vi "CI-recieveStatus.vi"(8 "error in (no error)":errorcluster, 10 "status":T1, 11 "common-interface in":refnum<class "VG-VNA_GUI.lvclass">) -> (0 "error out":errorcluster, 3 "common-interface out":refnum<class "VG-VNA_GUI.lvclass">)   [LabVIEW 2020, in "VG-VNA_GUI.lvlib" / "VG-VNA_GUI.lvclass"]
uses:
  VG-VNA_GUI.lvclass
  common/interface/CI-common_interface/CI-status_clust.ctl
  common/interface/CI-common_interface/CI-module_enum.ctl
  common/interface/CI-common_interface/CI-common_interface.lvclass
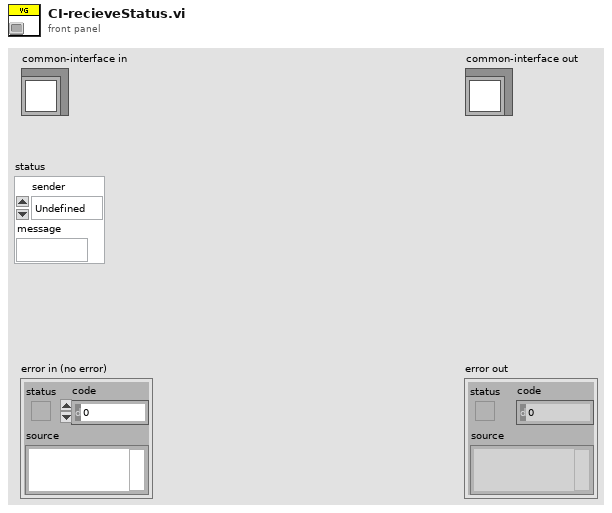
[diagram p1: front panel]
types:
  T1 = typedef "CI-common_interface.lvlib/CI-common_interface.lvclass/CI-status_clust.ctl" = cluster{"sender":T2, "message":string}
  T2 = typedef "CI-common_interface.lvlib/CI-common_interface.lvclass/CI-module_enum.ctl" = enum16{"Undefined", "HWM", "VDH", "GUI"}
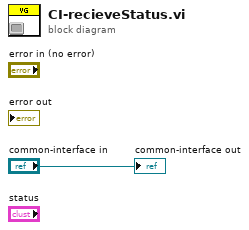
[diagram p0: block diagram]
diagram:
  "common-interface out" <- "common-interface in"
